vi "Data viewer.vi"(10 "data names":string[](array[string]), 11 "data cluster":cluster{"all data":dbl[][]}[](array[cluster])) -> ()   [LabVIEW 2020]
panel:
  in  "stop":bool
  out "Datasets":cluster{"xy data":dbl[][], "String":string}[](array[cluster])
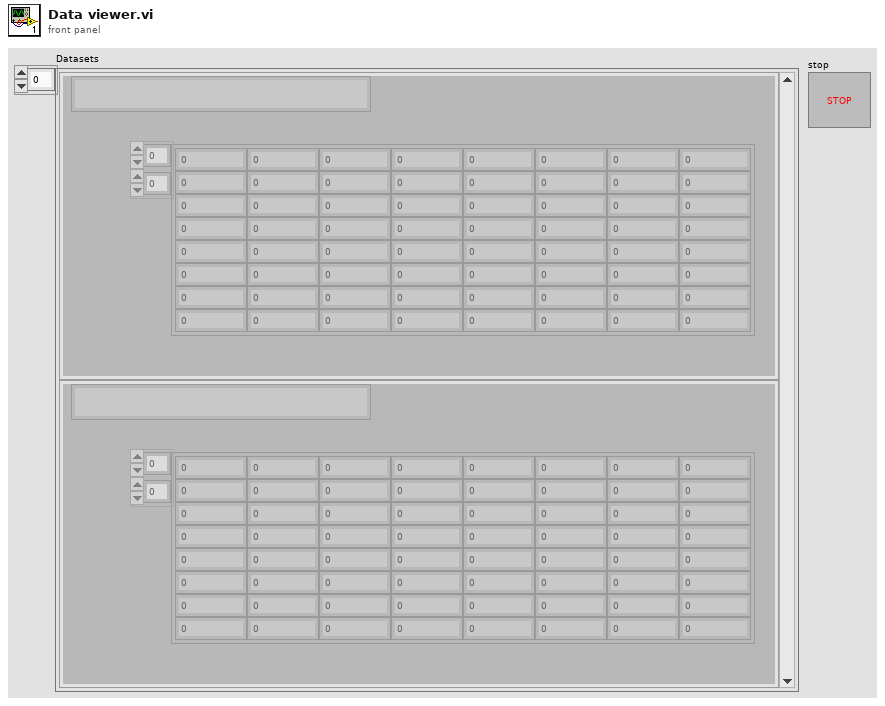
[diagram p1: front panel]
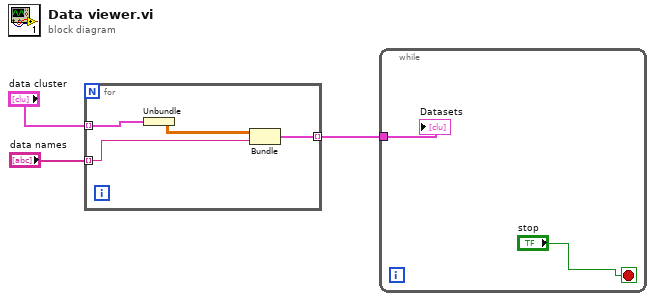
[diagram p0: block diagram]
diagram:
  n1 = for {
    tunnel: "data cluster" -> [w7] mode=indexing
    tunnel: "data names" -> [w5] mode=indexing
    tunnel: [w4] -> w1 mode=indexing
    n2 = Unbundle(w7) -> ("all data"=w6:dbl[][])
    n3 = Bundle("all data"=w6, w5) -> (w4:cluster{"all data":dbl[][], string})  [unwired: 1 in]
  }
  n4 = while {
    tunnel: w1 -> [w8]
    stop <- "stop" stop-if-true
    "Datasets" <- w8
  }
